vi "Get Slope and Offset.vi"(6 "Calibration Type":string, 7 "Position":u32, 8 "error in (no error)":errorcluster, 9 "DSpic Measurements":dbl[](array[numeric]), 10 "Measurements":dbl[](array[numeric]), 11 "Calibration in":refnum<class "Calibration.lvclass">) -> (0 "error out":errorcluster, 1 "Offset":dbl format="%#.3f", 2 "Scalar":dbl format="%#.3f", 3 "Calibration out":refnum<class "Calibration.lvclass">)   [LabVIEW 2015, in "Calibration.lvclass"]
uses:
  Calibration.lvclass
  <vilib>/Cree, Inc/Cree Test Framework/Core Launcher/Core Manager Methods -- Enum.ctl
  CBTF Applications/Driver Board Testing/Main/Application/Application/Class/Driver Board Test.lvclass
  <vilib>/Analysis/NI_AALPro.lvlib
  <vilib>/Cree, Inc/Cree Test Framework/Core Launcher/Core Launcher.lvlib
  <vilib>/Cree, Inc/Cree Test Framework/Classes/Data/Data Repo/Class/Data Repo.lvclass
  Classes/Application/Class/Application.lvclass
  Test Class/Test Class.lvclass
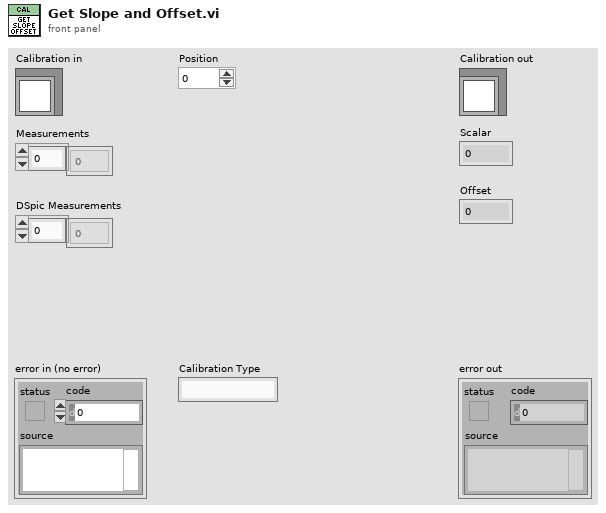
[diagram p1: front panel]
types:
  T1 = typedef "Core Launcher.lvlib/Core Manager Methods -- Enum.ctl" = enum16{"Spawn Objects", "Get Objects", "Destroy Objects"}
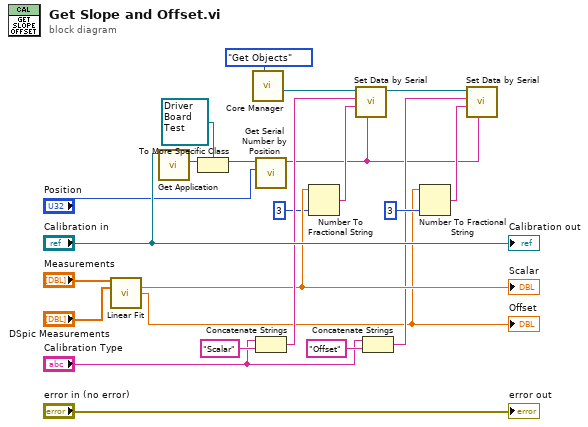
[diagram p0: block diagram]
diagram:
  n1 = call <vilib>:"Linear Fit.vi"("Y"="Measurements", "X"="DSpic Measurements") -> ("slope"=w9:dbl, "intercept"=w2:dbl)  [unwired: 9 in, 3 out]
  "Scalar" <- w9
  "Offset" <- w2
  n2 = call "Get Application.vi"("Test Class in"="Calibration in") -> ("Application.lvlib:Application.lvclass"=w18:refnum<class "Application.lvclass">)  [unwired: 9 in, 1 out]
  n3 = To More Specific Class(target class=refnum<class "Driver Board Test.lvclass"> refnum ("Driver Board Test in"), reference=w18) -> (specific class reference=w16:refnum<class "Driver Board Test.lvclass">)  [unwired: 1 in, 1 out]
  n4 = call <vilib>:"Core Manager.vi"("Method"=Core_Manager_Methods_--_Enum."Get Objects") -> ("Data Repo"=w14:refnum<class "Data Repo.lvclass">)  [unwired: 6 in, 4 out]
  n5 = call "Get Serial Number by Position.vi"("Position"="Position", "Application.lvclass"=w16) -> ("Value"=w3:string)  [unwired: 9 in]
  n6 = Concatenate Strings("Calibration Type", "Scalar" ("string")) -> (w10:string)
  n7 = Number To Fractional String(number=w9, precision (6)=i16 3 ("width (-)")) -> (F-format string=w8:string)  [unwired: 2 in]
  n8 = call <vilib>:"Set Data by Serial.vi"("Serial"=w3, "Value"=w8, "Header"=w10, "Acrobat Template in"=w14) -> ("Acrobat Template out"=w1:refnum<class "Data Repo.lvclass">)  [unwired: 6 in, 1 out]
  n9 = Concatenate Strings("Calibration Type", "Offset" ("string")) -> (w4:string)
  n10 = Number To Fractional String(number=w2, precision (6)=i16 3 ("width (-)")) -> (F-format string=w5:string)  [unwired: 2 in]
  n11 = call <vilib>:"Set Data by Serial.vi"("Serial"=w3, "Value"=w5, "Header"=w4, "Acrobat Template in"=w1) -> ()  [unwired: 6 in, 2 out]
  "error out" <- "error in (no error)"
  "Calibration out" <- "Calibration in"
